vi "Create Skipped.vi"(4 "Stack Trace":string, 5 "Test Case in":refnum<class "Test Case.lvclass">, 6 "Message":string, 8 "error in (no error)":errorcluster, 9 "Time":dbl, 10 "Classname":string, 11 "Name":string) -> (0 "error out":errorcluster, 3 "Test Case":refnum<class "Test Case.lvclass">)   [LabVIEW 2013, in "JUnit XML.lvlib" / "Test Case.lvclass"]
doc: "Creates a new instance of the <B>Test Case</B> class that represents a skipped test."
uses:
  Test Case.lvclass
  Test Result.ctl
  Test Case.lvclass/Test Case.ctl
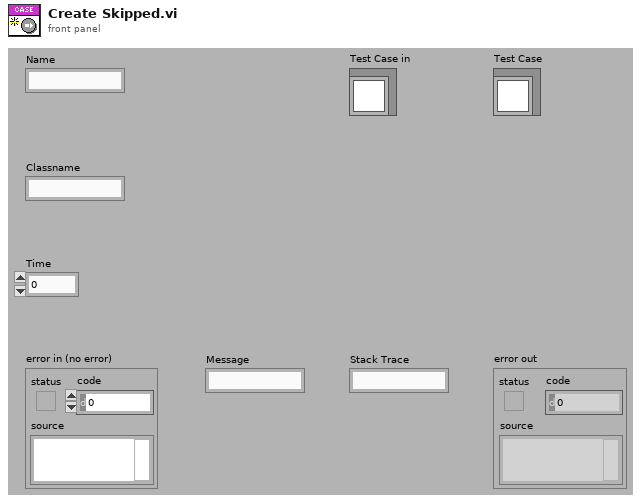
[diagram p1: front panel]
types:
  T1 = typedef "JUnit XML.lvlib/Test Case.lvclass/Test Result.ctl" = enum16{"Success", "Failure", "Error", "Skipped"}
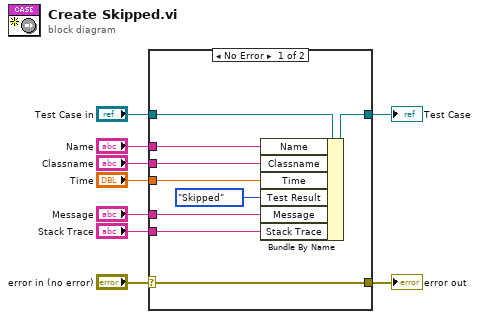
[diagram p0: block diagram]
diagram:
  n1 = case shown="No Error" "error in (no error)" {
    selector: "error in (no error)" -> [w18 w20]
    tunnel: [w18 w20] -> w8
    tunnel: [w16 w19] -> w6
    tunnel: "Test Case in" -> [w17 w19]
    tunnel: "Name" -> [w15 _]
    tunnel: "Classname" -> [w14 _]
    tunnel: "Time" -> [w13 _]
    tunnel: "Message" -> [w11 _]
    tunnel: "Stack Trace" -> [w10 _]
    frame No Error {
      n2 = Bundle By Name(cluster=w17, "Name"=w15, "Classname"=w14, "Time"=w13, "Test Result"=Test_Result."Skipped", "Message"=w11, "Stack Trace"=w10) -> (w16:refnum<class "Test Case.lvclass">)
    }
    frame Error {
    }
  }
  "error out" <- w8
  "Test Case" <- w6
